vi "报警交互入队列.vi"(8 "错误输入（无错误）":errorcluster, 9 "告警内容":string, 10 "告警码":string, 11 "报警模块":string) -> (0 "错误输出":errorcluster)   [LabVIEW 2016, in "Alarm interface.lvlib"]
uses:
  Alarm interface.lvlib
panel:
  out "输出簇":T1
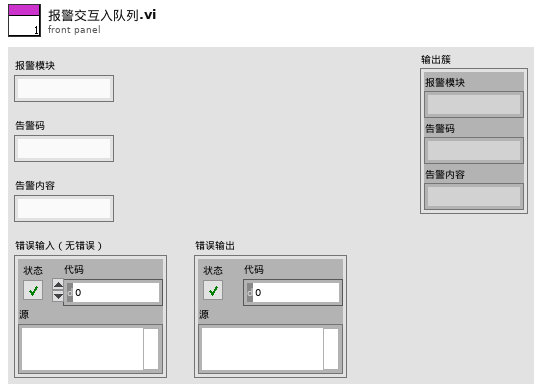
[diagram p1: front panel]
types:
  T1 = cluster{"报警模块":string, "告警码":string, "告警内容":string}
  T2 = cluster{"一级告警":string[][], "二级告警":string[][], "三级告警":string[][]}
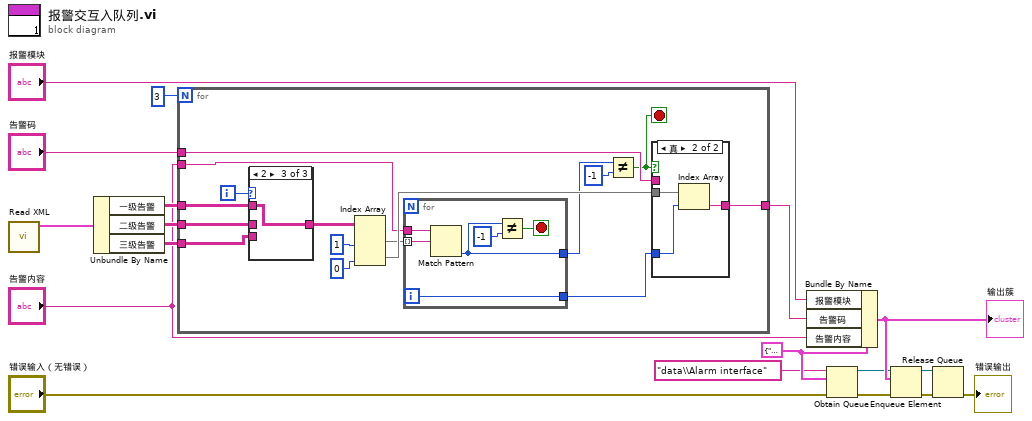
[diagram p0: block diagram]
diagram:
  w16 = T1 {"报警模块"="", "告警码"="", "告警内容"=""}
  n1 = call "Read XML.vi"() -> ("值"=w8:T2)  [unwired: 10 in, 1 out]
  n2 = Unbundle By Name(w8) -> ("一级告警"=w7:string[][], "二级告警"=w6:string[][], "三级告警"=w5:string[][])
  n3 = for {
    N: 3 -> [_]
    tunnel: "告警内容" -> [w29]
    tunnel: "告警码" -> [w28]
    tunnel: [w25] -> w1
    tunnel: w7 -> [w24]
    tunnel: w6 -> [w23]
    tunnel: w5 -> [w22]
    i -> [w27]
    stop <- w26 stop-if-true
    n4 = case shown="2" w27 {
      tunnel: [w41 w42 w43] -> w33
      tunnel: w24 -> [_ _ w43]
      tunnel: w23 -> [_ w42 _]
      tunnel: w22 -> [w41 _ _]
      frame 0, Default {
      }
      frame 1 {
      }
      frame 2 {
      }
    }
    n5 = Index Array(array=w33, index (col) #1=1 ("禁用的索引 (列)"), index (col) #2=0 ("索引 (列)")) -> (element #1=w20:string[], element #2=w30:string[])  [unwired: 2 in]
    n6 = for {
      tunnel: w29 -> [w36]
      tunnel: [w38] -> w21
      tunnel: w20 -> [w37] mode=indexing
      tunnel: [w35] -> w19
      i -> [w35]
      stop <- w39 stop-if-true
      n7 = Match Pattern(string=w36, regular expression=w37) -> (offset past match=w38:i32)  [unwired: 1 in, 3 out]
      n8 = Not Equal?(x=w38, y=-1) -> (x != y?=w39:bool)
    }
    n9 = Not Equal?(x=w21, y=-1) -> (x != y?=w26:bool)
    n10 = case shown="真" w26 {
      tunnel: w30 -> [_ w47]
      tunnel: w19 -> [_ w46]
      tunnel: [w44 w45] -> w25
      tunnel: w28 -> [w44 _]
      frame False {
      }
      frame True {
        n11 = Index Array(array=w47, index=w46) -> (element=w45:string)
      }
    }
  }
  n12 = Bundle By Name(cluster=w16, "报警模块"="报警模块", "告警码"=w1, "告警内容"="告警内容") -> (w17:T1)
  "输出簇" <- w17
  n13 = Obtain Queue(name (unnamed)="data\\Alarm interface" ("名称（未命名）"), element data type=w16, error in (no error)="错误输入（无错误）") -> (queue out=w12:refnum<queue>, error out=w13:errorcluster)  [unwired: 2 in, 1 out]
  n14 = Enqueue Element(queue=w12, element=w17, error in (no error)=w13) -> (queue out=w14:refnum<queue>, error out=w15:errorcluster)  [unwired: 1 in, 1 out]
  n15 = Release Queue(queue=w14, error in (no error)=w15) -> (error out=→"错误输出":errorcluster)  [unwired: 1 in, 2 out]
